vi "CCE RRMA P04 SubVI04.vi"(11 "entrada neurona":dbl[](array[numeric])=[0.9997525383124077, 0.022047103684425993, 0.00047771658598479535, 0.0029255984598577215, 8.143259107920102e-07, 4.0976510303173995e-06, -2.948715981189433e-07]) -> (3 "element":string)   [LabVIEW 2020]
doc: "Ceballos Conde Emanuel Rodríguez Ramírez Miguel Ángel 4MV6 Sistemas de visión artificial 2022/1\nEste vi contiene el funcionamiento de una neurona compet y a su vez la memoria que esta requiere para operar, este vi da como resultado el nombre del objeto en memoria que detecte la neurona respecto a la entrada"
panel:
  out "logical OR":bool
  out "min value":dbl
  out "Array":dbl[](array[numeric])
  out "appended array":dbl[][](array[numeric])
  # "Ceballos Conde Emanuel\nRodríguez Ramírez Miguel Ángel\n4MV6\nSistemas de visión artificial\n2022/1"
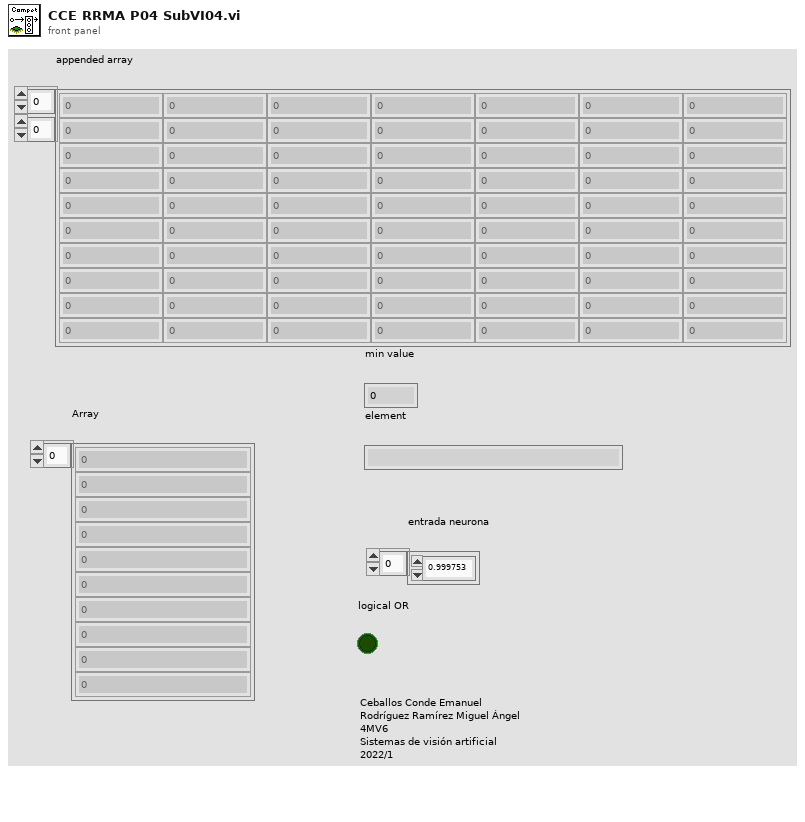
[diagram p1: front panel]
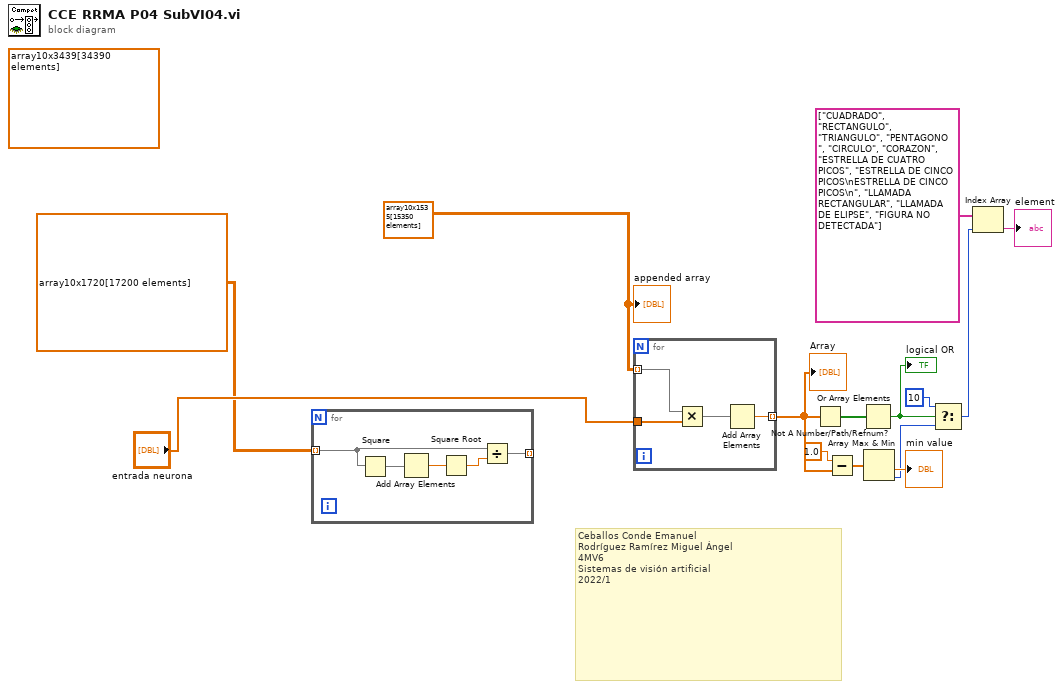
[diagram p0: block diagram]
diagram:
  w3 = dbl[][] array10x1535[15350 elements] ("Rxx")
  (unwired) dbl[][] array10x3439[34390 elements] ("Rxx")
  # "Ceballos Conde Emanuel\nRodríguez Ramírez Miguel Ángel\n4MV6\nSistemas de visión artificial\n2022/1"
  n1 = for {
    tunnel: dbl[][] array10x1720[17200 elements] ("normalizado") -> [w16] mode=indexing
    tunnel: [w15] -> _ mode=indexing
    n2 = Square(x=w16) -> (x^2=w18:dbl[])
    n3 = Add Array Elements(numeric array=w18) -> (sum=w19:dbl)
    n4 = Square Root(x=w19) -> (sqrt(x)=w17:dbl)
    n5 = Divide(x=w16, y=w17) -> (x/y=w15:dbl[])
  }
  n6 = for {
    tunnel: w3 -> [w23] mode=indexing
    tunnel: "entrada neurona" -> [w22]
    tunnel: [w20] -> w10 mode=indexing
    n7 = Multiply(x=w23, y=w22) -> (x*y=w21:dbl[])
    n8 = Add Array Elements(numeric array=w21) -> (sum=w20:dbl)
  }
  "Array" <- w10
  n9 = Not A Number/Path/Refnum?(number/path/refnum=w10) -> (NaN/Path/Refnum?=w8:bool[])
  n10 = Subtract(x=1.0, y=w10) -> (x-y=w13:dbl[])
  n11 = Or Array Elements(Boolean array=w8) -> (logical OR=w9:bool)
  "logical OR" <- w9
  n12 = Array Max & Min(array=w13) -> (min value=→"min value":dbl, min index (indices)=w6:i32)  [unwired: 2 out]
  n13 = Select(t=10, s=w9, f=w6) -> (s? t:f=w7:i32)
  n14 = Index Array(array=string[] ["CUADRADO", "RECTANGULO", "TRIANGULO", "PENTAGONO ", "CIRCULO", "CORAZON", "ESTRELLA DE CUATRO PICOS", "ESTRELLA DE CINCO PICOS\nESTRELLA DE CINCO PICOS\n", "LLAMADA RECTANGULAR", "LLAMADA DE ELIPSE", "FIGURA NO DETECTADA"], index=w7) -> (element=→"element":string)
  "appended array" <- w3
